vi "ParameterSweepCore.vi"(4 "Round Trip":bool, 6 "Initialize":bool, 7 "Backward in":bool, 8 "Step":dbl, 9 "Stop":dbl, 10 "Start":dbl, 11 "Value in":dbl) -> (0 "New Sweep":bool, 1 "Total Steps":dbl, 3 "Value out":dbl, 5 "Backward out":bool)   [LabVIEW 2020]
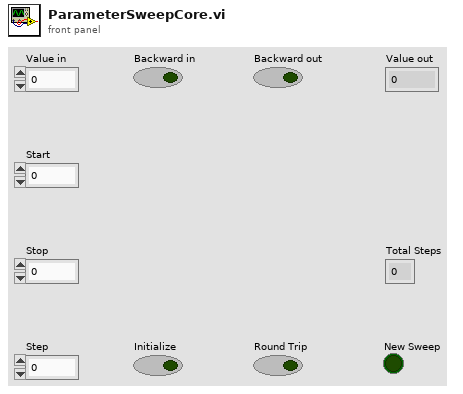
[diagram p1: front panel]
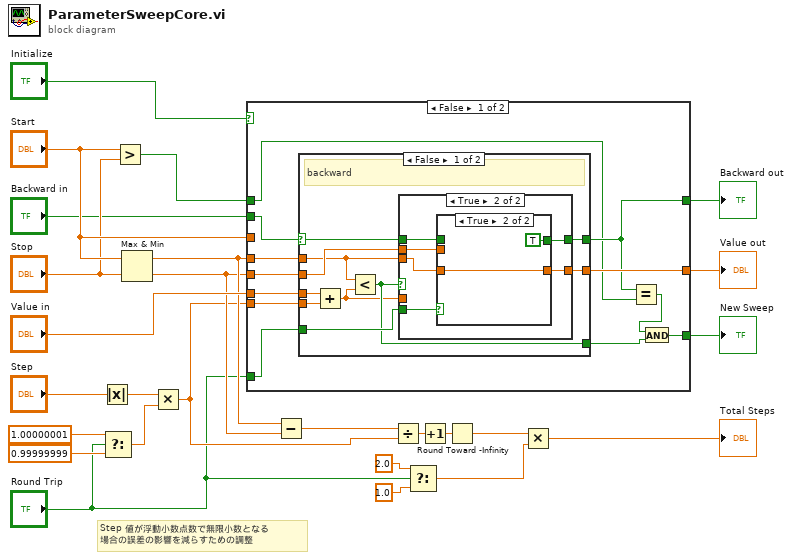
[diagram p0: block diagram]
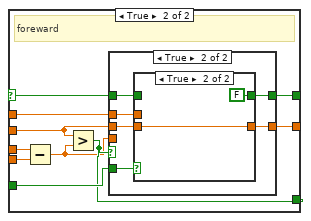
[diagram p4: hidden frame]
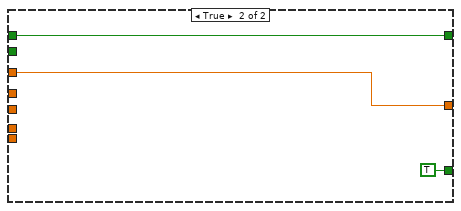
[diagram p7: hidden frame]
diagram:
  # "Step 値が浮動小数点数で無限小数となる\n場合の誤差の影響を減らすための調整"
  n1 = Absolute Value(x="Step") -> (abs(x)=w17:dbl)
  n2 = Select(t=1.00000001 ("y"), s="Round Trip", f=0.99999999 ("y")) -> (s? t:f=w13:dbl)
  n3 = Greater?(x="Start", y="Stop") -> (0:w23:bool)
  n4 = Max & Min(x="Start", y="Stop") -> (max(x,y)=w9:dbl, min(x,y)=w8:dbl)
  n5 = Multiply(x=w17, y=w13) -> (x*y=w7:dbl)
  n6 = case shown="False" "Initialize" {
    tunnel: "Value in" -> [w37 _]
    tunnel: "Backward in" -> [w31 _]
    tunnel: "Start" -> [_ w85]
    tunnel: [w35 w85] -> w25
    tunnel: w23 -> [w27 w84]
    tunnel: [w32 w84] -> w24
    tunnel: w7 -> [w38 _]
    tunnel: w9 -> [w36 _]
    tunnel: w8 -> [w34 _]
    tunnel: "Round Trip" -> [w33 _]
    tunnel: [w28 TRUE] -> w16
    frame False {
      n7 = case shown="False" w31 {
        selector: w31 -> [w46 w66]
        tunnel: w38 -> [w48 w69]
        tunnel: w37 -> [w47 w70]
        tunnel: w36 -> [w40 w64]
        tunnel: [w45 w67] -> w32
        tunnel: [w44 w68] -> w35
        tunnel: w34 -> [w42 w61]
        tunnel: w33 -> [w43 w65]
        tunnel: [w41 w63] -> w29
        frame False {
          # "backward"
          n8 = Add(x=w47, y=w48) -> (x+y=w39:dbl)
          n9 = Less?(x=w40, y=w39) -> (x < y?=w41:bool)
          n10 = case shown="True" w41 {
            tunnel: [w50 w56] -> w45
            tunnel: w46 -> [w50 w51]
            tunnel: w39 -> [w49 _]
            tunnel: [w49 w54] -> w44
            tunnel: w40 -> [_ w55]
            tunnel: w43 -> [_ w53]
            tunnel: w42 -> [_ w52]
            frame False {
            }
            frame True {
              n11 = case shown="True" w53 {
                tunnel: [w57 TRUE] -> w56
                tunnel: w55 -> [_ w59]
                tunnel: [w58 w59] -> w54
                tunnel: w52 -> [w58 _]
                tunnel: w51 -> [w57 _]
                frame False {
                }
                frame True {
                }
              }
            }
          }
        }
        frame True {
          # "foreward"
          n12 = Subtract(x=w70, y=w69) -> (x-y=w62:dbl)
          n13 = Greater?(x=w61, y=w62) -> (0:w63:bool)
          n14 = case shown="True" w63 {
            tunnel: w61 -> [_ w76]
            tunnel: [w72 w77] -> w68
            tunnel: [w71 w78] -> w67
            tunnel: w62 -> [w72 _]
            tunnel: w66 -> [w71 w74]
            tunnel: w65 -> [_ w75]
            tunnel: w64 -> [_ w73]
            frame False {
            }
            frame True {
              n15 = case shown="True" w75 {
                tunnel: [w80 FALSE] -> w78
                tunnel: [w79 w81] -> w77
                tunnel: w76 -> [_ w81]
                tunnel: w74 -> [w80 _]
                tunnel: w73 -> [w79 _]
                frame False {
                }
                frame True {
                }
              }
            }
          }
        }
      }
      n16 = Equal?(x=w32, y=w27) -> (x = y?=w30:bool)
      n17 = And(x=w30, y=w29) -> (x .and. y?=w28:bool)
    }
    frame True {
    }
  }
  "Value out" <- w25
  "Backward out" <- w24
  "New Sweep" <- w16
  n18 = Subtract(x=w9, y=w8) -> (x-y=w11:dbl)
  n19 = Divide(x=w11, y=w7) -> (x/y=w10:dbl)
  n20 = Select(t=2.0, s="Round Trip", f=1.0) -> (s? t:f=w2:dbl)
  n21 = Increment(x=w10) -> (x+1=w12:dbl)
  n22 = Round Toward -Infinity(1:w12) -> (0:w3:dbl)
  n23 = Multiply(x=w3, y=w2) -> (x*y=→"Total Steps":dbl)
